vi "ToAddress.vi"(1 "Input":u8) -> (0 "Address":T1)   [LabVIEW 2016]
uses:
  DataTypes/Addresses.ctl
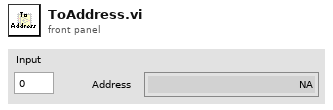
[diagram p1: front panel]
types:
  T1 = typedef "Addresses.ctl" = enum8{"NA", "Slot1/AI0-AccelerometerAx", "Slot1/AI1-AccelerometerAz", "Slot1/AI2-AccelerometerBy", "Slot1/AI3-AccelerometerBz", "Slot2/AI0-AccelerometerCx", "Slot2/AI1-AccelerometerCz", "Slot2/AI2-AccelerometerDy", "Slot2/AI3-AccelerometerDz", "Slot3/DIO0-ModbusSubnetATx", "Slot3/DIO1-ModbusSubnetBTx", "Slot3/DIO2-ModbusSubnetCTx", "Slot3/DIO3-ModbusSubnetDTx", "Slot3/DIO4-ModbusSubnetARx", "Slot3/DIO5-ModbusSubnetBRx", "Slot3/DIO6-ModbusSubnetCRx", "Slot3/DIO7-ModbusSubnetDRx", "Slot4/DIO0-ModbusSubnetETx", "Slot4/DIO1-GyroTx", "Slot4/DIO2", "Slot4/DIO3", "Slot4/DIO4-ModbusSubnetERx", "Slot4/DIO5-GyroRx", "Slot4/DIO6", "Slot4/DIO7", "Slot5/DI0-ILCPowerInterlockStatus", "Slot5/DI1-FanCoilHeaterInterlockStatus", "Slot5/DI2-LaserTrackerInterlockStatus", "Slot5/DI3-AirSupplyInterlockStatus", "Slot5/DI4-GISEarthquakeInterlockStatus", "Slot5/DI5-GISEStopInterlockStatus", "Slot5/DI6-TMAMotionStopInterlockStatus", "Slot5/DI7-GISHeartbeatInterlockStatus", "Slot5/DI8-AirSupplyValveOpen", "Slot5/DI9-AirSupplyValveClosed", "Slot5/DI10-MirrorCellLightsOn", "Slot5/DI11", "Slot5/DI12", "Slot5/DI13", "Slot5/DI14", "Slot5/DI15", "Slot5/DO0", "Slot5/DO1", "Slot5/DO2", "Slot5/DO3", "Slot5/DO4", "Slot5/DO5", "Slot5/DO6", "Slot5/DO7", "Slot5/DO8", "Slot5/DO9", "Slot5/DO10", "Slot5/DO11", "Slot5/DO12", "Slot5/DO13", "Slot5/DO14", "Slot5/DO15", "Slot6/CH0-HeartbeatToSafetyController", "Slot6/CH1-CriticalFaultToSafetyController", "Slot6/CH2-MirrorLoweringRaisingToSafetyController", "Slot6/CH3-MirrorParkedToSafetyController", "Slot6/CH4-AirSupplyValveControl", "Slot6/CH5-MirrorCellLightControl", "Slot6/CH6", "Slot6/CH7", "Slot7/CH0", "Slot7/CH1", "Slot7/CH2", "Slot7/CH3", "Slot7/CH4", "Slot7/CH5", "Slot7/CH6", "Slot7/CH7", "Slot8/Port1-Displacement", "Slot8/Port2-Inclinometer", "Slot8/Port3", "Slot8/Port4", "Undefined1", "Undefined2", "Undefined3", "Undefined4", "Undefined5", "Undefined6", "Undefined7", "Undefined8", "Undefined9", "Undefined10", "Undefined11", "Undefined12", "Undefined13", "Undefined14", "Undefined15", "Undefined16", "Undefined17", "Undefined18", "Undefined19", "Undefined20", "Undefined21", "Undefined22", "Undefined23", "Undefined24", "Undefined25", "Undefined26", "Undefined27", "Undefined28", "Undefined29", "Undefined30", "Undefined31", "Undefined32", "Undefined33", "Undefined34", "Undefined35", "Undefined36", "Undefined37", "Undefined38", "Undefined39", "Undefined40", "Undefined41", "Undefined42", "Undefined43", "Undefined44", "Undefined45", "Undefined46", "Undefined47", "Undefined48", "Undefined49", "Undefined50", "Undefined51", "Undefined52", "Undefined53", "Undefined54", "Undefined55", "Undefined56", "Undefined57", "Undefined58", "Undefined59", "Undefined60", "Undefined61", "Undefined62", "Undefined63", "Undefined64", "Undefined65", "Undefined66", "Undefined67", "Undefined68", "Undefined69", "Undefined70", "Undefined71", "Undefined72", "Undefined73", "Undefined74", "Undefined75", "Undefined76", "Undefined77", "Undefined78", "Undefined79", "Undefined80", "Undefined81", "Undefined82", "Undefined83", "Undefined84", "Undefined85", "Undefined86", "Undefined87", "Undefined88", "Undefined89", "Undefined90", "Undefined91", "Undefined92", "Undefined93", "Undefined94", "Undefined95", "Undefined96", "Undefined97", "Undefined98", "Undefined99", "Undefined100", "Undefined101", "Undefined102", "Undefined103", "Undefined104", "Undefined105", "Undefined106", "Undefined107", "Undefined108", "Undefined109", "Undefined110", "Undefined111", "Undefined112", "Undefined113", "Undefined114", "Undefined115", "Undefined116", "Undefined117", "Undefined118", "Undefined119", "Undefined120", "Undefined121", "Undefined122", "Undefined123", "Undefined124", "Undefined125", "Undefined126", "Undefined127", "Undefined128", "Undefined129", "Undefined130", "Undefined131", "Undefined132", "Undefined133", "Undefined134", "Undefined135", "Undefined136", "Undefined137", "Undefined138", "Undefined139", "Undefined140", "Undefined141", "Undefined142", "Undefined143", "Undefined144", "Undefined145", "Undefined146", "Undefined147", "Undefined148", "Undefined149", "Undefined150", "Undefined151", "Undefined152", "Undefined153", "Undefined154", "Undefined155", "Undefined156", "Undefined157", "Undefined158", "Undefined159", "Undefined160", "Undefined161", "Undefined162", "Undefined163", "Undefined164", "Undefined165", "Undefined166", "Undefined167", "Undefined168", "Undefined169", "Undefined170", "Undefined171", "Undefined172", "Undefined173", "Undefined174", "Undefined175", "ModbusSoftwareTrigger", "Accelerometers", "HealthAndStatus", "Timestamp"}
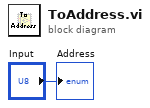
[diagram p0: block diagram]
diagram:
  "Address" <- "Input"
